vi "DAE_Query.vi"(0 "System no.":i32=1 min=1 max=4 step=1, 2 "Axes to query":string[](array[string]), 3 "All axes?":bool, 4 "Axis identifier?":bool=TRUE, 5 "error in":errorcluster) -> (14 "DDL Error":i32[](array[numeric]), 19 "error out":errorcluster)   [LabVIEW 2020]
doc: "Returns DDL autoexamined error. See GCS DLL manual for details.\n\nE-710: Only supported by 6-channel version. Only one axis per command allowed. \"All axes\" must be FALSE. Only valid for axes for which the autoexamine function has been enabled using DAS.vi."
panel:
  # "Returns DDL autoexamined error. See GCS DLL manual for details."
  # "If all axes: use"
  # "Query"
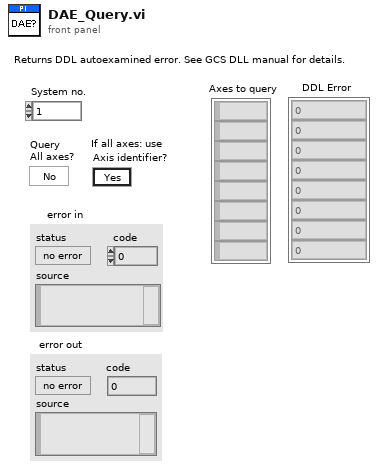
[diagram p1: front panel]
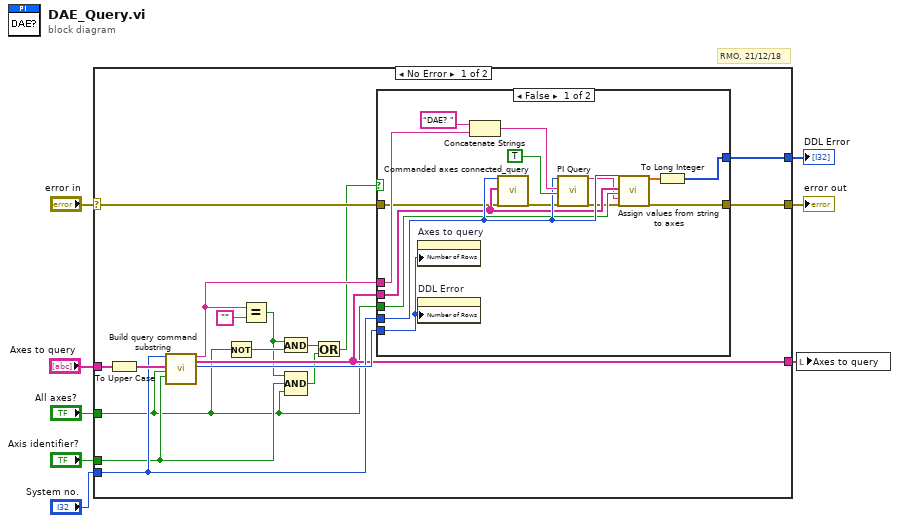
[diagram p0: block diagram]
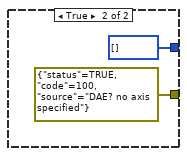
[diagram p2: hidden frame]
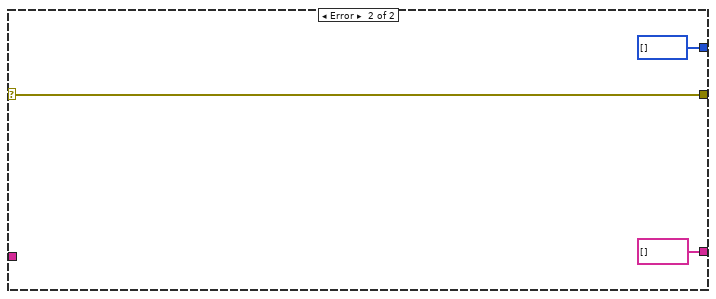
[diagram p3: hidden frame]
diagram:
  # "RMO, 21/12/18"
  n1 = case shown="No Error" "error in" {
    selector: "error in" -> [w11 w44]
    tunnel: [w25 i32[] []] -> w8
    tunnel: "Axes to query" -> [w24 _]
    tunnel: [w10 w44] -> w6
    tunnel: "System no." -> [w19 _]
    tunnel: [w18 string[] [] ("Axes to query out")] -> w4
    tunnel: "Axis identifier?" -> [w14 _]
    tunnel: "All axes?" -> [w13 _]
    frame No Error {
      n2 = To Upper Case(1:w24) -> (0:w22:string[])
      n3 = call "Build query command substring.vi"("System no."=w19, "Axes to query in"=w22, "Query\nAll axes?"=w13, "For all axes: use\nAxis identifier?"=w14) -> ("Command substring"=w21:string, "Axes to query out"=w18:string[], "Number of rows"=w20:u32)  [unwired: 2 in, 11 out]
      n4 = Not(x=w13) -> (.not. x?=w17:bool)
      n5 = Equal?(x=w21, y="" ("x")) -> (x = y?=w15:bool)
      n6 = And(x=w15, y=w17) -> (x .and. y?=w16:bool)
      n7 = Compound Arithmetic op=AND(w15, w14, w13) -> (w12:bool)
      n8 = Or(x=w16, y=w12) -> (x .or. y?=w9:bool)
      n9 = case shown="False" w9 {
        tunnel: [w26 i32[] []] -> w25
        tunnel: w21 -> [w37 _]
        tunnel: w20 -> [w36 _]
        tunnel: w19 -> [w35 _]
        tunnel: w18 -> [w34 _]
        tunnel: w13 -> [w33 _]
        tunnel: w11 -> [w31 _]
        tunnel: [w30 errorcluster {"status"=TRUE, "code"=100, "source"="DAE? no axis specified"} ("error out")] -> w10
        frame False {
          n10 = property on="Axes to query" class="Arr (strict)"("Number of Rows"=w36) -> ()  [unwired: 2 in, 2 out]
          n11 = property on="DDL Error" class="Arr (strict)"("Number of Rows"=w36) -> ()  [unwired: 2 in, 2 out]
          n12 = Concatenate Strings("DAE? ", w37) -> (w38:string)
          n13 = call "Commanded axes connected_query.vi"("System no."=w35, "Commanded axes"=w34, "error in"=w31) -> ("error out"=w32:errorcluster)  [unwired: 1 in, 15 out]
          n14 = call "PI Query.vi"("System no."=w35, "String to send"=w38, "Attach termination char.?"=TRUE ("Attach Linefeed?"), "error in"=w32) -> ("String read"=w28:string, "error out"=w29:errorcluster)  [unwired: 3 in, 11 out]
          n15 = call "Assign values from string to axes.vi"("System no."=w35, "Queried axes"=w34, "All axes queried?"=w33, "Input String"=w28, "error in"=w29) -> ("Values"=w27:dbl[], "error out"=w30:errorcluster)  [unwired: 4 in, 9 out]
          n16 = To Long Integer(number=w27) -> (32bit integer=w26:i32[])
        }
        frame True {
        }
      }
    }
    frame Error {
    }
  }
  "error out" <- w6
  "DDL Error" <- w8
  n17 = local write "Axes to query"(w4) -> ()
